vi "VoltageInput Sensor Event Example.vi"() -> ()   [LabVIEW 2012, in "Phidget Voltage Input.lvlib"]
uses:
  <instrlib>/Phidgets/Phidget Voltage Input/Phidget Voltage Input.lvlib
  <instrlib>/Phidgets/Phidget Voltage Input/Public/VoltageInputStart.vi
  <instrlib>/Phidgets/Phidget Voltage Input/Public/VoltageInputClose.vi
  <instrlib>/Phidgets/Phidget Common/Phidget Common.lvlib
panel:
  out "Unit Name":string
  out "Unit Symbol":string
  in  "Sensor Type":u32(ring) items=["SENSOR_TYPE_VOLTAGE"=0, "SENSOR_TYPE_1114"=11140, "SENSOR_TYPE_1117"=11170, "SENSOR_TYPE_1123"=11230, "SENSOR_TYPE_1127"=11270, "SENSOR_TYPE_1130_PH"=11301, "SENSOR_TYPE_1130_ORP"=11302, "SENSOR_TYPE_1132"=11320, "SENSOR_TYPE_1133"=11330, "SENSOR_TYPE_1135"=11350, "SENSOR_TYPE_1142"=11420, "SENSOR_TYPE_1143"=11430, "SENSOR_TYPE_3500"=35000, "SENSOR_TYPE_3501"=35010, "SENSOR_TYPE_3502"=35020, "SENSOR_TYPE_3503"=35030, "SENSOR_TYPE_3507"=35070, "SENSOR_TYPE_3508"=35080, "SENSOR_TYPE_3509"=35090, "SENSOR_TYPE_3510"=35100, "SENSOR_TYPE_3511"=35110, "SENSOR_TYPE_3512"=35120, "SENSOR_TYPE_3513"=35130, "SENSOR_TYPE_3514"=35140, "SENSOR_TYPE_3515"=35150, "SENSOR_TYPE_3516"=35160, "SENSOR_TYPE_3517"=35170, "SENSOR_TYPE_3518"=35180, "SENSOR_TYPE_3519"=35190, "SENSOR_TYPE_3584"=35840, "SENSOR_TYPE_3585"=35850, "SENSOR_TYPE_3586"=35860, "SENSOR_TYPE_3587"=35870, "SENSOR_TYPE_3588"=35880, "SENSOR_TYPE_3589"=35890, "SENSOR_TYPE_ADP1000_PH"=110000, "SENSOR_TYPE_ADP1000_ORP"=110001]
  in  "IsHubPort":bool
  out "Sensor Value":dbl caption="Voltage" format="%.2f"
  in  "stop":bool
  out "Serial Number Return":i32
  in  "Device Info":T1={"Serial Number"=-1, "Channel"=0, "Port"=0}
  out "error out":errorcluster
  # "Be sure to use this stop button to stop the program.\nIf you use the \"Abort Execution\" button, you will\nneed to use PhidgetResetLibrary.vi or restart Labview \nin order for any Phidgets to work."
  # "Yes\n\nNo"
  # "Be sure to set sensor type to the sensor you're using.\nNo SensorChange events will fire using\nSENSOR_TYPE_VOLTAGE"
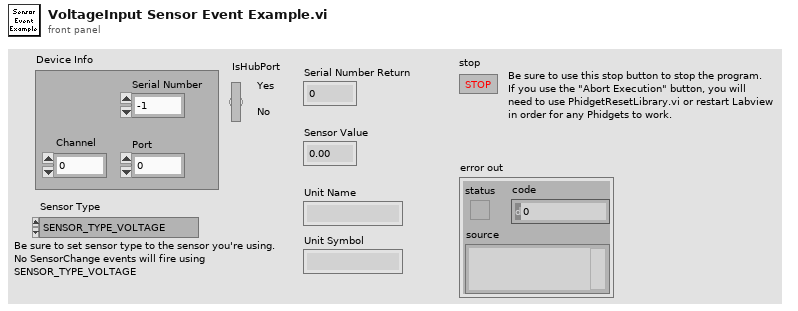
[diagram p1: front panel]
types:
  T1 = cluster{"Serial Number":i32, "Channel":i32, "Port":i32}
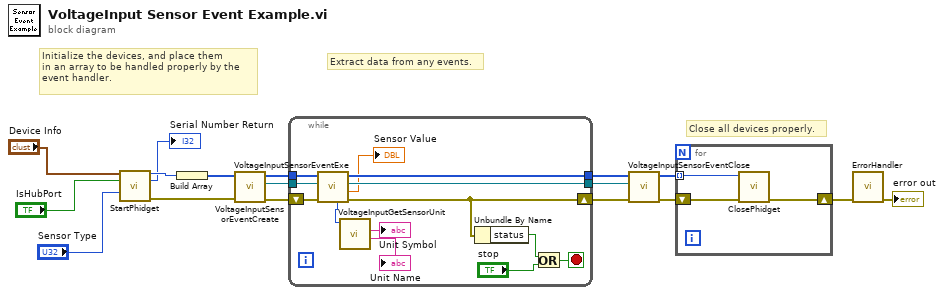
[diagram p0: block diagram]
diagram:
  # "Close all devices properly."
  # "Extract data from any events."
  # "Initialize the devices, and place them\nin an array to be handled properly by the\nevent handler."
  n1 = call-poly <instrlib>:"StartPhidget.vi"("Device Info"="Device Info", "IsHubPort"="IsHubPort", "Sensor Type"="Sensor Type") -> ("Phidget ID"=w7:u64, "Serial Number Return"=→"Serial Number Return":i32, "error out"=w2:errorcluster)  [unwired: 9 in, 1 out]
  n2 = Build Array(w7) -> (w17:u64[])
  n3 = call <instrlib>:"VoltageInputSensorEventCreate.vi"("error in (no error)"=w2, "Devices In"=w17) -> ("error out"=w10:errorcluster, "Event Registration Refnum"=w15:refnum<event-registration>, "Devices Out"=w16:u64[])  [unwired: 7 in]
  n4 = while {
    tunnel: w16 -> [w30]
    tunnel: w15 -> [w26]
    tunnel: [w29] -> w12
    shift-right: [w25] -> w11
    shift-left: w10 -> [w28]
    tunnel: [w27] -> w5
    stop <- w24 stop-if-true
    n5 = call <instrlib>:"VoltageInputSensorEventExe.vi"("error in (no error)"=w28, "Event Registration Refnum In"=w26, "Devices In"=w30) -> ("error out"=w25:errorcluster, "Sensor Value"=→"Sensor Value":dbl, "Event Registration Refnum Out"=w29:refnum<event-registration>, "Devices Out"=w27:u64[], "phid"=w20:u64)  [unwired: 2 in, 2 out]
    n6 = call <instrlib>:"VoltageInputGetSensorUnit.vi"("Device In"=w20) -> ("Name"=→"Unit Name":string, "Symbol"=→"Unit Symbol":string)  [unwired: 6 in, 2 out]
    n7 = Unbundle By Name(w25) -> ("status"=w22:bool)
    n8 = Or(x=w22, y="stop") -> (x .or. y?=w24:bool)
  }
  n9 = call <instrlib>:"VoltageInputSensorEventClose.vi"("error in (no error)"=w11, "Event Registration Refnum In"=w12, "Devices In"=w5) -> ("error out"=w8:errorcluster, "Devices Out"=w6:u64[])  [unwired: 7 in]
  n10 = for {
    tunnel: w6 -> [w31] mode=indexing
    shift-right: [w33] -> w14
    shift-left: w8 -> [w32]
    n11 = call-poly <instrlib>:"ClosePhidget.vi"("error in"=w32, "Device In"=w31) -> ("error out"=w33:errorcluster)  [unwired: 9 in]
  }
  n12 = call <instrlib>:"ErrorHandler.vi"("error in"=w14) -> ("error out"=→"error out":errorcluster)  [unwired: 9 in, 1 out]
